vi "predefined to Cell row [ ].vi"(1 "Predefined Borders":T20={"Borders"=0, "Header"={"Thickness"=1.0, "Line"=0, "Background "=16777226}, "Data"={"Thickness"=0.5, "Line"=0, "Background "=16777215}}, 2 "Titles or datas":T19, 5 "Format Column Header or Data":T18, 7 "Row Header?":bool, 9 "Format Row Header":T18, 11 "error in (no error)":errorcluster, 12 "Title tous":T10[][](array[typedef]), 13 "Header Column size":cluster{"# Column":u16, "# Row":u16}, 14 "Table size":cluster{"# Column":u16, "# Row":u16}) -> (8 "Row  [ ]":T1, 15 "error duplicate":errorcluster)   [LabVIEW 2019, in "Exaprom PDF.lvlib" / "Pdfp Table Class.lvclass"]
doc: "Version 2.0\nDeveloped by Jean-Marc Simard\nCopyright © 2012, Exaprom Inc.\nAll rights reserved.\nLicense: BSD\n\nWith iTextSharp 4.1.6 (http://itextsharp.sourceforge.net)\nunder Mozilla Public License Version 1.1\n(http://www.mozilla.org/MPL/MPL-1.1.html)"
uses:
  Pdfp Table Class.lvclass
  Controls/Table Controls/Row Predefined borders cluster.ctl
  Controls/Table Controls/Row Predefined borders.ctl
  Controls/Table Controls/Cell Font, type, Alignment and LS V2.ctl
  Controls/Table Controls/Cell Type, Alignment and LS.ctl
  Controls/Table Controls/Cell Alignment 20px.ctl
  Controls/Table Controls/Text vertical arrangement.ctl
  Controls/Text Controls/Line spacing.ctl
  Controls/Font Controls/Font complete cluster.ctl
  Controls/Font Controls/Font size.ctl
  Controls/Font Controls/Font color.ctl
  Controls/Font Controls/Type and encoding.ctl
  Controls/Text Controls/Unicode/Type and run direction.ctl
  Controls/Table Controls/Table Custom type Titles or Datas.ctl
  Controls/Table Controls/Cell Border 20 px.ctl
  Controls/Table Controls/Table Appearance and Font Row [ ].ctl
  Controls/Table Controls/One Row Appearance.ctl
  Controls/Table Controls/Row from to.ctl
  Controls/Table Controls/Cell, Alignment, LS and Font - hide Vmerge.ctl
  Controls/Table Controls/Cell Appearance.ctl
  Controls/Table Controls/Merge Horizontal.ctl
  Controls/Table Controls/Merge Vertical.ctl
  Controls/Table Controls/Cell, Alignment, LS and Font.ctl
  Exaprom PDF.lvlib
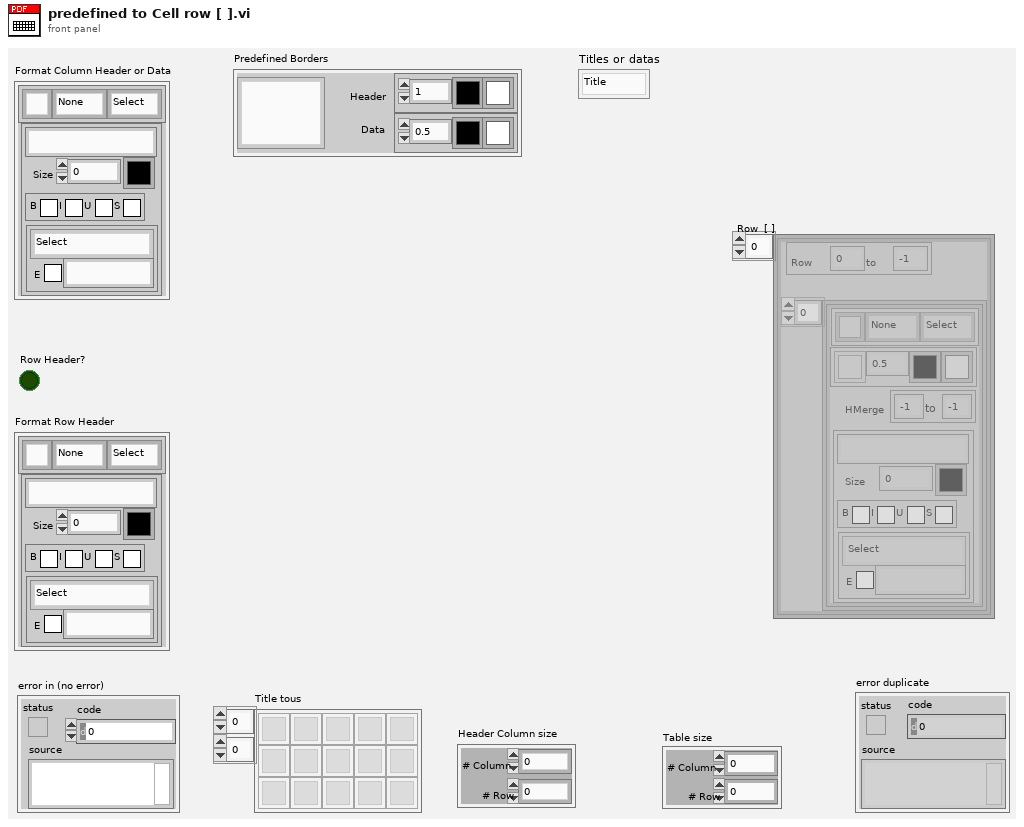
[diagram p1: front panel]
types:
  T1 = typedef "Exaprom PDF.lvlib/Table Appearance and Font Row [ ].ctl" = T2[]
  T2 = typedef "Exaprom PDF.lvlib/One Row Appearance.ctl" = cluster{"Row":T3, "Cell [ ]":T4[]}
  T3 = typedef "Exaprom PDF.lvlib/Row from to.ctl" = cluster{"From #":i16, "to #":i16}
  T4 = typedef "Exaprom PDF.lvlib/Cell, Alignment, LS and Font - hide Vmerge.ctl" = cluster{"Text":T5, "Cell Appearance":T9, "HMerge":T11, "VMerge":T12, "Font":T13}
  T5 = typedef "Exaprom PDF.lvlib/Cell Type, Alignment and LS.ctl" = cluster{"Cell Alignment":T6, "Text rotation":T7, "Line spacing":T8}
  T6 = typedef "Exaprom PDF.lvlib/Cell Alignment 20px.ctl" = u16
  T7 = typedef "Exaprom PDF.lvlib/Text vertical arrangement.ctl" = enum16{"None", "Clockwise", "Counterclockwise"}
  T8 = typedef "Exaprom PDF.lvlib/Line spacing.ctl" = enum16{"Select", "1.0", "1.5", "2.0"}
  T9 = typedef "Exaprom PDF.lvlib/Cell Appearance.ctl" = cluster{"Border":T10, "Thickness":sgl, "Color":u32, "BG":u32}
  T10 = typedef "Exaprom PDF.lvlib/Cell Border 20 px.ctl" = u16
  T11 = typedef "Exaprom PDF.lvlib/Merge Horizontal.ctl" = cluster{"From":i8, "to":i8}
  T12 = typedef "Exaprom PDF.lvlib/Merge Vertical.ctl" = cluster{"From":i8, "to":i8}
  T13 = typedef "Exaprom PDF.lvlib/Font complete cluster.ctl" = cluster{"Name":string, "Size":T14, "Color":T15, "Style":cluster{"Bold":bool, "Italic":bool, "Underline":bool, "Strikeout":bool}, "Type":T16}
  T14 = typedef "Exaprom PDF.lvlib/Font size.ctl" = sgl
  T15 = typedef "Exaprom PDF.lvlib/Font color.ctl" = u32
  T16 = typedef "Exaprom PDF.lvlib/Type and encoding.ctl" = cluster{"Type&direction":T17, "Embedded":bool, "Encoding":string}
  T17 = typedef "Exaprom PDF.lvlib/Type and run direction.ctl" = enum16{"Select", "ASCII", "UTF-16", "UTF-16 (default)", "UTF-16 (LTR)", "UTF-16 (RTL)"}
  T18 = typedef "Exaprom PDF.lvlib/Cell Font, type, Alignment and LS V2.ctl" = cluster{"Cell Type, Alignment and LS":T5, "Font":T13}
  T19 = typedef "Exaprom PDF.lvlib/Table Custom type Titles or Datas.ctl" = enum16{"Title", "Data"}
  T20 = typedef "Exaprom PDF.lvlib/Row Predefined borders cluster.ctl" = cluster{"Borders":T21, "Header":cluster{"Thickness":sgl, "Line":u32, "Background ":u32}, "Data":cluster{"Thickness":sgl, "Line":u32, "Background ":u32}}
  T21 = typedef "Exaprom PDF.lvlib/Row Predefined borders.ctl" = u16
  T22 = typedef "Exaprom PDF.lvlib/Cell, Alignment, LS and Font.ctl" = cluster{"Text":T5, "Cell Appearance":T9, "HMerge":T11, "VMerge":T12, "Font":T13}
  T23 = cluster{cluster{"# Row":u16, "# Row":u16}, T22[]}[]
  T24 = cluster{cluster{"# Row":u16, "# Row":u16}, T22[]}
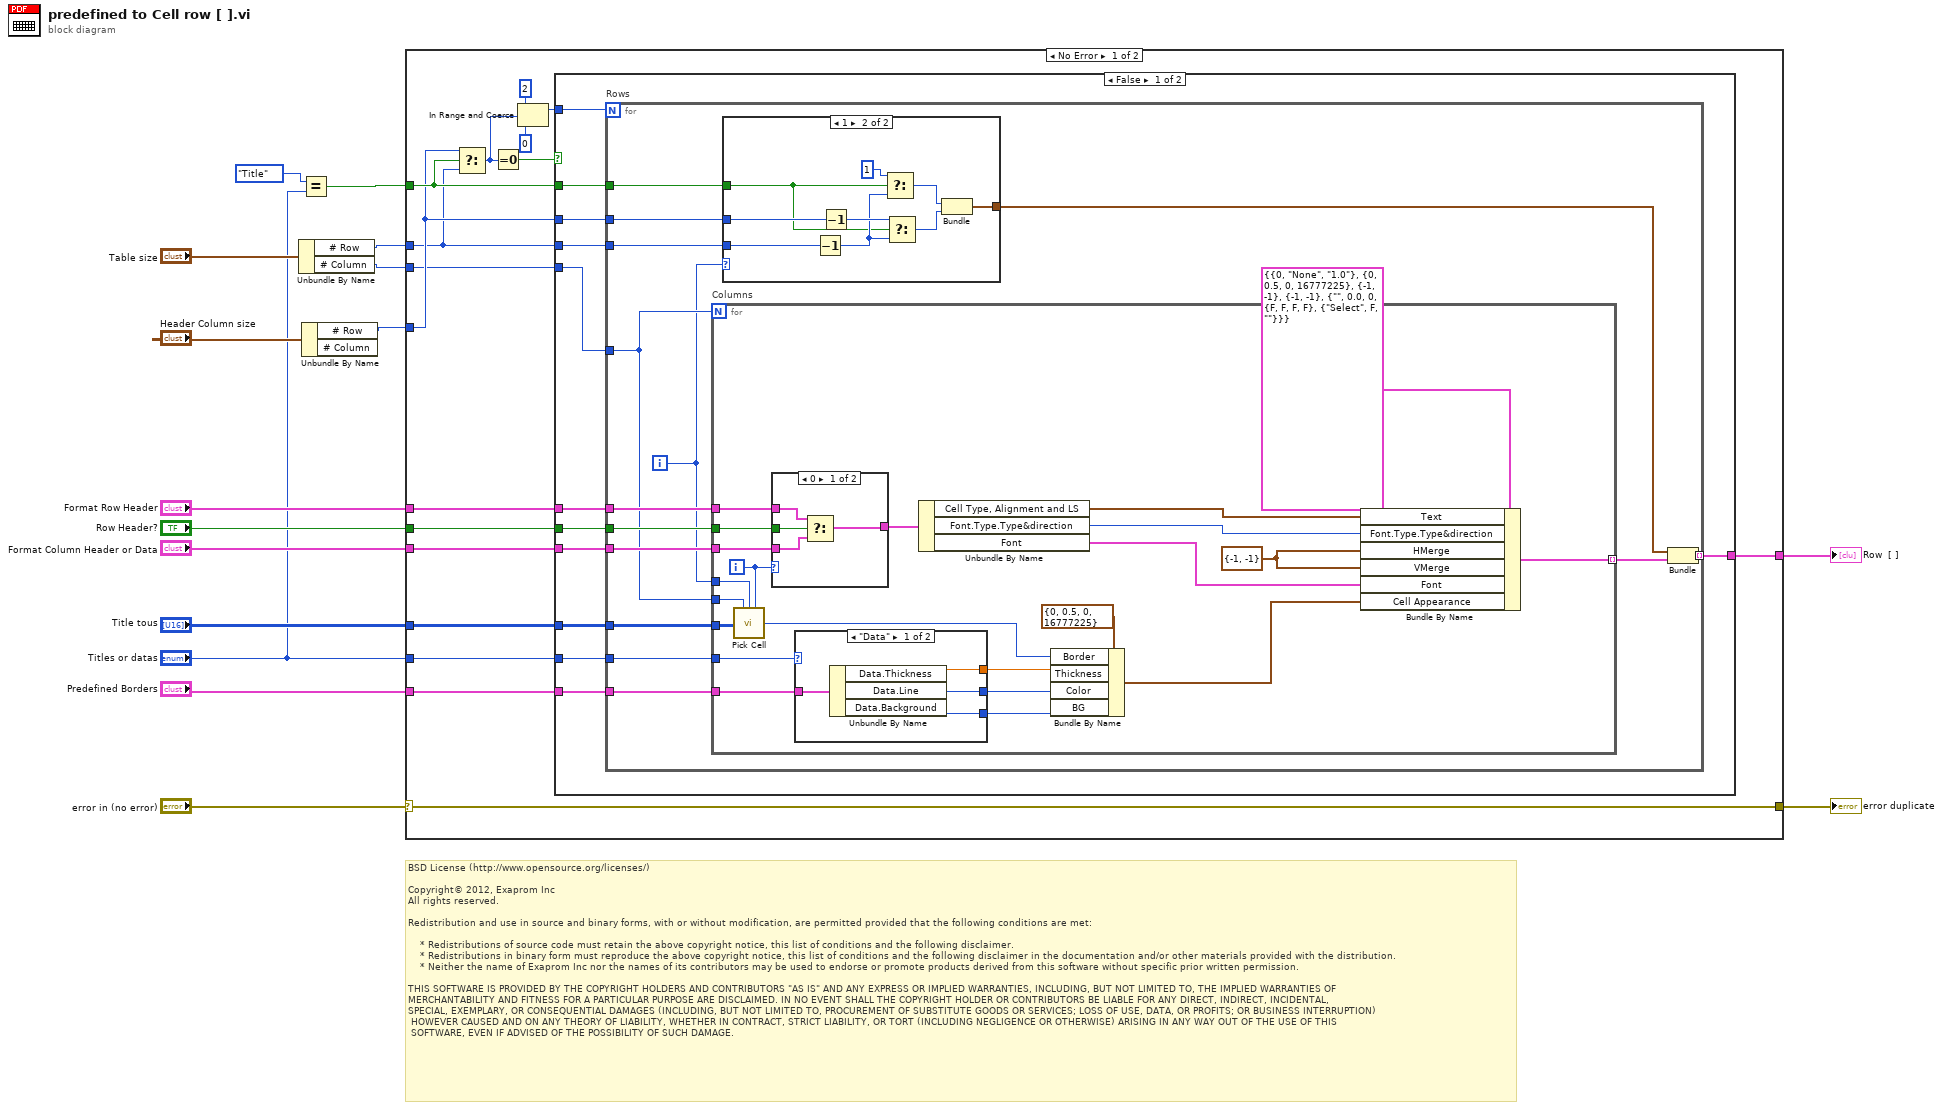
[diagram p0: block diagram]
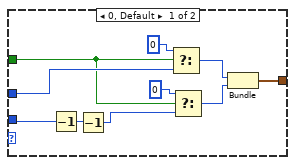
[diagram p2: hidden frame]
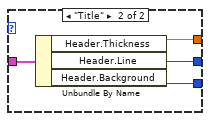
[diagram p4: hidden frame]
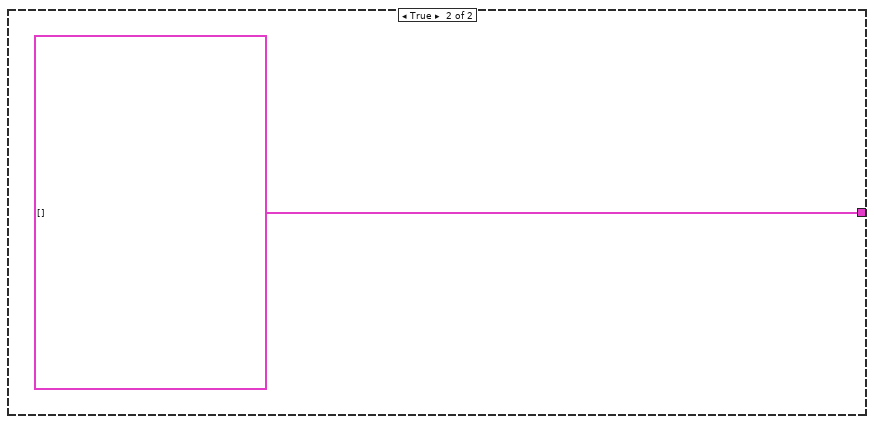
[diagram p5: hidden frame]
diagram:
  # "BSD License (http://www.opensource.org/licenses/)\n\nCopyright© 2012, Exaprom Inc\nAll rights reserved.\n\nRedistribution and use in source and binary forms, with or without modification, are permitted provided that the following conditions are met:\n\n    * Redistributions of source code must retain the above copyright notice, this list of conditions and the following disclaimer.\n    * Redistributions in binary form must reproduce the above copyright notice, this list of conditions and the following disclaimer in the documentation and/or other materials provided with the distribution.\n    * Neither the name of Exaprom Inc nor the names of its contributors may be used to endorse or promote products derived from this software without specific prior written permission.\n\nTHIS SOFTWARE IS PROVIDED BY THE COPYRIGHT HOLDERS AND CONTRIBUTORS \"AS IS\" AND ANY EXPRESS OR IMPLIED WARRANTIES, INCLUDING, BUT NOT LIMITED TO, THE IMPLIED WARRANTIES OF \nMERCHANTABILITY AND FITNESS FOR A PARTICULAR PURPOSE ARE DISCLAIMED. IN NO EVENT SHALL THE COPYRIGHT HOLDER OR CONTRIBUTORS BE LIABLE FOR ANY DIRECT, INDIRECT, INCIDENTAL,\nSPECIAL, EXEMPLARY, OR CONSEQUENTIAL DAMAGES (INCLUDING, BUT NOT LIMITED TO, PROCUREMENT OF SUBSTITUTE GOODS OR SERVICES; LOSS OF USE, DATA, OR PROFITS; OR BUSINESS INTERRUPTION)\n HOWEVER CAUSED AND ON ANY THEORY OF LIABILITY, WHETHER IN CONTRACT, STRICT LIABILITY, OR TORT (INCLUDING NEGLIGENCE OR OTHERWISE) ARISING IN ANY WAY OUT OF THE USE OF THIS\n SOFTWARE, EVEN IF ADVISED OF THE POSSIBILITY OF SUCH DAMAGE."
  n1 = Unbundle By Name("Table size") -> ("# Row"=w4:u16, "# Column"=w1:u16)
  n2 = Equal?(x=Table_Custom_type_Titles_or_Datas."Title" ("Titles or datas"), y="Titles or datas") -> (x = y?=w6:bool)
  n3 = Unbundle By Name("Header Column size") -> ("# Row"=w5:u16)  [unwired: 1 out]
  n4 = case shown="No Error" "error in (no error)" {
    selector: "error in (no error)" -> [w33 w115]
    tunnel: [w33 w115] -> w16
    tunnel: "Predefined Borders" -> [w32 _]
    tunnel: [w31 _] -> w3
    tunnel: "Format Row Header" -> [w29 _]
    tunnel: "Titles or datas" -> [w30 _]
    tunnel: "Row Header?" -> [w28 _]
    tunnel: "Format Column Header or Data" -> [w27 _]
    tunnel: "Title tous" -> [w26 _]
    tunnel: w6 -> [w25 _]
    tunnel: w5 -> [w24 _]
    tunnel: w4 -> [w23 _]
    tunnel: w1 -> [w21 _]
    frame No Error {
      n5 = Select(t=w24, s=w25, f=w23) -> (s? t:f=w20:u16)
      n6 = Equal To 0?(x=w20) -> (x = 0?=w22:bool)
      n7 = In Range and Coerce(upper limit=u16 2, x=w20, lower limit=u16 0) -> (coerced(x)=w17:u16)  [unwired: 1 out]
      n8 = case shown="False" w22 {
        tunnel: w32 -> [w45 _]
        tunnel: [w44 T23 []] -> w31
        tunnel: w30 -> [w43 _]
        tunnel: w29 -> [w42 _]
        tunnel: w28 -> [w41 _]
        tunnel: w27 -> [w40 _]
        tunnel: w26 -> [w39 _]
        tunnel: w25 -> [w38 _]
        tunnel: w24 -> [w37 _]
        tunnel: w23 -> [w36 _]
        tunnel: w21 -> [w35 _]
        tunnel: w17 -> [w34 _]
        frame False {
          n9 = for "Rows" {
            N: w34 -> [_]
            tunnel: w45 -> [w59]
            tunnel: [w51] -> w44 mode=indexing
            tunnel: w35 -> [w53]
            tunnel: w43 -> [w58]
            tunnel: w42 -> [w57]
            tunnel: w41 -> [w56]
            tunnel: w40 -> [w55]
            tunnel: w39 -> [w54]
            tunnel: w38 -> [w48]
            tunnel: w37 -> [w47]
            tunnel: w36 -> [w46]
            i -> [w50]
            n10 = for "Columns" {
              N: w53 -> [_]
              tunnel: w57 -> [w87]
              tunnel: w59 -> [w100]
              tunnel: w58 -> [w99]
              tunnel: w56 -> [w88]
              tunnel: w55 -> [w86]
              tunnel: w54 -> [w84]
              tunnel: w53 -> [w82]
              tunnel: w50 -> [w80]
              tunnel: [w79] -> w52 mode=indexing
              i -> [w81]
              w90 = T11 {"From"=-1, "to"=-1} ("HMerge")
              n11 = call "Pick Cell.vi"("# Column"=w82, "i Row"=w80, "i Column"=w81, "Title tous"=w84) -> ("Cell border"=w83:T10)  [unwired: 11 in]
              n12 = case shown="0" w81 {
                tunnel: w88 -> [w104 _]
                tunnel: w87 -> [w103 _]
                tunnel: w86 -> [w102 w105]
                tunnel: [w101 w105] -> w85
                frame 0 {
                  n13 = Select(t=w103, s=w104, f=w102) -> (s? t:f=w101:T18)
                }
                frame 1.., Default {
                }
              }
              n14 = case shown="\"Data\"" w99 {
                tunnel: w100 -> [w109 w113]
                tunnel: [w108 w112] -> w95
                tunnel: [w107 w111] -> w94
                tunnel: [w106 w110] -> w93
                frame "Data" {
                  n15 = Unbundle By Name(w109) -> ("Data.Thickness"=w108:sgl, "Data.Line"=w107:u32, "Data.Background"=w106:u32)
                }
                frame "Title" {
                  n16 = Unbundle By Name(w113) -> ("Header.Thickness"=w112:sgl, "Header.Line"=w111:u32, "Header.Background"=w110:u32)
                }
              }
              n17 = Unbundle By Name(w85) -> ("Cell Type, Alignment and LS"=w97:T5, "Font.Type.Type&direction"=w92:T17, "Font"=w89:T13)
              n18 = Bundle By Name(cluster=T9 {"Border"=0, "Thickness"=0.5, "Color"=0, "BG"=16777225} ("Cell Appearance"), "Border"=w83, "Thickness"=w95, "Color"=w94, "BG"=w93) -> (w91:T9)
              n19 = Bundle By Name(cluster=T22 {"Text"={"Cell Alignment"=0, "Text rotation"=enum."None", "Line spacing"=enum."1.0"}, "Cell Appearance"={"Border"=0, "Thickness"=0.5, "Color"=0, "BG"=16777225}, "HMerge"={"From"=-1, "to"=-1}, "VMerge"={"From"=-1, "to"=-1}, "Font"={"Name"="", "Size"=0.0, "Color"=0, "Style"={"Bold"=FALSE, "Italic"=FALSE, "Underline"=FALSE, "Strikeout"=FALSE}, "Type"={"Type&direction"=enum."Select", "Embedded"=FALSE, "Encoding"=""}}} ("Cell, Alignment, LS and Font"), "Text"=w97, "Font.Type.Type&direction"=w92, "HMerge"=w90, "VMerge"=w90, "Font"=w89, "Cell Appearance"=w91) -> (w79:T22)
            }
            n20 = case shown="1" w50 {
              tunnel: [w69 w78] -> w49
              tunnel: w48 -> [w60 w70]
              tunnel: w47 -> [w64 w73]
              tunnel: w46 -> [w63 w74]
              frame 0, Default {
                n21 = Decrement(x=w63) -> (x-1=w62:u16)
                n22 = Decrement(x=w62) -> (x-1=w61:u16)
                n23 = Select(t=u16 0 ("# Row"), s=w60, f=w64) -> (s? t:f=w67:u16)
                n24 = Select(t=u16 0 ("# Row"), s=w60, f=w61) -> (s? t:f=w65:u16)
                n25 = Bundle("# Row"=w67, "# Row"=w65) -> (w69:cluster{"# Row":u16, "# Row":u16})  [unwired: 1 in]
              }
              frame 1 {
                n26 = Decrement(x=w74) -> (x-1=w71:u16)
                n27 = Decrement(x=w73) -> (x-1=w72:u16)
                n28 = Select(t=u16 1 ("# Row"), s=w70, f=w71) -> (s? t:f=w76:u16)
                n29 = Select(t=w72, s=w70, f=w71) -> (s? t:f=w75:u16)
                n30 = Bundle("# Row"=w76, w75) -> (w78:cluster{"# Row":u16, u16})  [unwired: 1 in]
              }
            }
            n31 = Bundle(w49, w52) -> (w51:T24)  [unwired: 1 in]
          }
        }
        frame True {
        }
      }
    }
    frame Error {
    }
  }
  "error duplicate" <- w16
  "Row  [ ]" <- w3
